vi "TDMS List Field Value From All Runs.vi"(8 "error in (no error)":errorcluster, 10 "Property Name":string, 11 "TDMS File Path":path) -> (0 "error out":errorcluster, 1 "Found?":bool, 2 "Property Values":string[](array[string]), 3 "TDMS File Path Out":path)   [LabVIEW 2011]
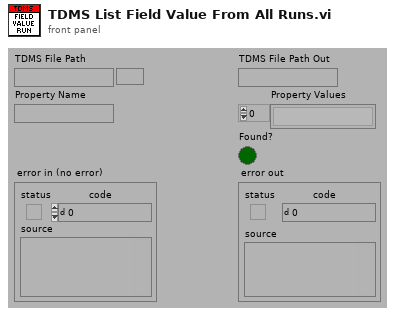
[diagram p1: front panel]
types:
  T1 = enum16{"open", "open or create", "create or replace", "create", "open (read-only)"}
  T2 = typedef "Connection Refnum.ctl" = cluster{"Environment Handle":i32, "Connection Handle":i32}
  T3 = typedef "Field Record.ctl" = cluster{"ixField":i32, "iSequenceOrder":i32, "sxFieldId":string, "sxSequenceId":string, "sDisplayName":string, "sValue":string, "sUnits":string, "nDataType":T4, "nNextItem":T5, "fSystem":bool, "fSystemValue":bool, "fRequired":bool, "fSetAtTest":bool, "fTestField":bool, "fDeleted":bool, "fIndexed":bool, "fFreeList":bool}
  T4 = typedef "Field DataTypes.ctl" = enum32{"text", "numeric", "list", "timestamp", "boolean"}
  T5 = typedef "Field NextItem.ctl" = enum32{"Reset", "Retain", "Auto-Increment"}
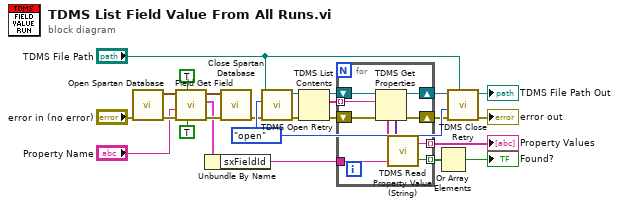
[diagram p0: block diagram]
diagram:
  w24 = T1."open" ("operation (0:open)")
  n1 = call "Open Spartan Database.vi"("error in (no error)"="error in (no error)") -> ("error out"=w14:errorcluster, "Connection Refnum"=w13:T2)  [unwired: 9 in]
  n2 = call "Field Get Field.vi"("by sDisplayName? (f, by sFieldId)"=TRUE, "Include deleted? (F)"=TRUE, "error in (no error)"=w14, "sFieldId or sDisplayName (\"\")"="Property Name", "Connection Refnum"=w13) -> ("error out"=w11:errorcluster, "Field"=w6:T3, "Connection Refnum"=w12:T2)  [unwired: 3 in, 1 out]
  n3 = Unbundle By Name(w6) -> ("sxFieldId"=w4:string)
  n4 = call "Close Spartan Database.vi"("error in (no error)"=w11, "Connection Refnum"=w12) -> ("error out"=w9:errorcluster)  [unwired: 9 in]
  n5 = call "TDMS Open Retry.vi"("error in (no error)"=w9, "Operation (0:open)"=w24, "Path"="TDMS File Path") -> ("error out"=w23:errorcluster, "TDMS File Ref"=w21:refnum<k34>)  [unwired: 1 in, 6 out]
  n6 = TDMS List Contents(4:w23, 7:w21) -> (0:w22:errorcluster, 2:w19:string[], 3:w20:refnum<k34>)  [unwired: 1 in, 1 out]
  n7 = for {
    tunnel: w19 -> [w33] mode=indexing
    tunnel: w4 -> [w31]
    shift-right: [w30] -> w17
    shift-left: w22 -> [w35]
    shift-right: [w29] -> w18
    shift-left: w20 -> [w34]
    tunnel: [w28] -> w1 mode=indexing
    tunnel: [w26] -> w3 mode=indexing
    n8 = TDMS Get Properties(8:w35, 10:w33, 11:w34) -> (0:w30:errorcluster, 3:w29:refnum<k34>, 4:w32:variant[], 6:w27:string[])  [unwired: 3 in, 2 out]
    n9 = call "TDMS Read Property Value (String).vi"("Property Name"=w31, "Property Names"=w27, "Property Values"=w32) -> ("Found?"=w26:bool, "Property Value"=w28:string)
  }
  "Property Values" <- w1
  n10 = Or Array Elements(Boolean array=w3) -> (logical OR=→"Found?":bool)
  n11 = call "TDMS Close Retry.vi"("TDMS Path"="TDMS File Path", "error in (no error)"=w17, "Operation (0:open)"=w24, "TDMS File Ref"=w18) -> ("error out"=→"error out":errorcluster, "TDMS Path Out"=→"TDMS File Path Out":path)  [unwired: 1 in, 5 out]
